vi "Rotate WayPt after Arc.vi"(9 "Phantom Waypoint":cluster{"x":dbl, "y":dbl, "th":dbl}, 10 "Waypoint Line rad":dbl, 11 "Pt 0":cluster{"x":dbl, "y":dbl, "th":dbl}) -> (3 "Phantom Waypoint out":cluster{"x":dbl, "y":dbl, "th":dbl})   [LabVIEW 2018]
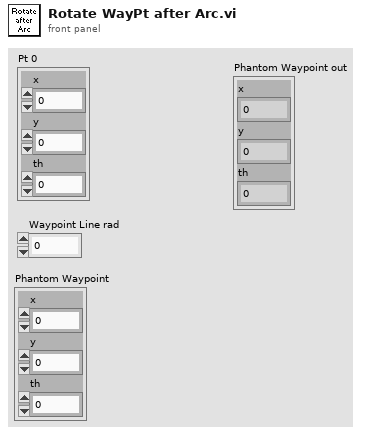
[diagram p1: front panel]
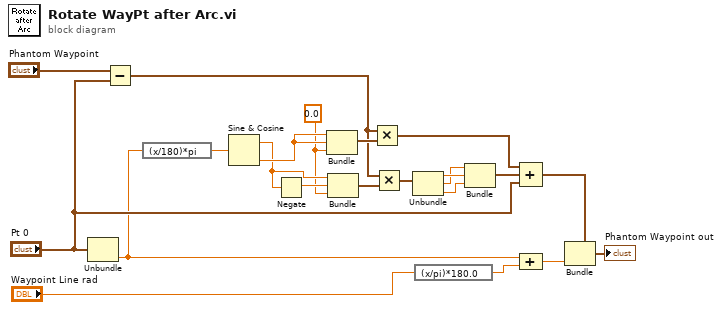
[diagram p0: block diagram]
diagram:
  w15 = 0.0
  n1 = Unbundle("Pt 0") -> ("th"=w2:dbl)  [unwired: 2 out]
  n2 = Subtract(x="Phantom Waypoint", y="Pt 0") -> (x-y=w13:cluster{"x":dbl, "y":dbl, "th":dbl})
  n3 = expression code="(x/180)*pi" ("radians to degrees")(w2) -> (w1:dbl)
  n4 = Sine & Cosine(0:w1) -> (1:w16:dbl, 2:w18:dbl)
  n5 = Negate(x=w16) -> (-x=w17:dbl)
  n6 = Bundle(w18, w18, w15) -> (w14:cluster{dbl, dbl, dbl})  [unwired: 1 in]
  n7 = Bundle(w16, w17, w15) -> (w12:cluster{dbl, dbl, dbl})  [unwired: 1 in]
  n8 = Multiply(x=w13, y=w14) -> (x*y=w6:cluster{dbl, dbl, dbl})
  n9 = Multiply(x=w13, y=w12) -> (x*y=w9:cluster{dbl, dbl, dbl})
  n10 = Unbundle(w9) -> (w11:dbl, w10:dbl, w8:dbl)
  n11 = expression code="(x/pi)*180.0" ("radians to degrees")("Waypoint Line rad") -> (w22:dbl)
  n12 = Bundle(w10, w11, w8) -> (w7:cluster{dbl, dbl, dbl})  [unwired: 1 in]
  n13 = Compound Arithmetic op=ADD(w6, w7, "Pt 0") -> (w4:cluster{dbl, dbl, dbl})
  n14 = Compound Arithmetic op=ADD(w2, w22) -> (w20:dbl)
  n15 = Bundle(cluster=w4, w20) -> (→"Phantom Waypoint out":cluster{dbl, dbl, dbl})  [unwired: 2 in]
